vi "Data entry form.vi"(0 "Stack in":refnum<class "Stack.lvclass">, 1 "Adhesive type":string, 2 "Temperature (C)":string, 3 "Relative humidity":string, 5 "Position":dbl, 7 "Module Type":string, 9 "Module?":bool, 11 "error in (no error)":errorcluster, 12 "Operator":string, 13 "ROC version":string) -> (4 "Stack out":refnum<class "Stack.lvclass">, 8 "Cancelled?":bool, 15 "error out":errorcluster)   [LabVIEW 2021, in "Stack.lvclass"]
uses:
  Stack.lvclass
  Stack.lvclass/Stack.ctl
panel:
  in  "?":string="If blank, name automatically assigned. Check DB after submission!!!"
  in  "(optional) Module stack name (no hyphens; include 320)":string
  in  "Cancel Button":bool
  in  "Comments":string
  in  "?":string="Leave Base/Top Layer ID fields empty for dummy runs!!"
  in  "?":string="Record sensor visual inspection comments here."
  out "Sensor thickness":string
  out "BP Type":string
  out "Geometry":string
  in  "Baselayer thickness for glue dispense":dbl
  out "Resolution":string
  out "Date":string
  in  "Glue Batch":string
  in  "Component Tray ID":string
  in  "Assembly Tray ID":string
  in  "PUT ID":string
  in  "Baselayer ID":string
  in  "Toplayer ID":string
  in  "Submit":bool
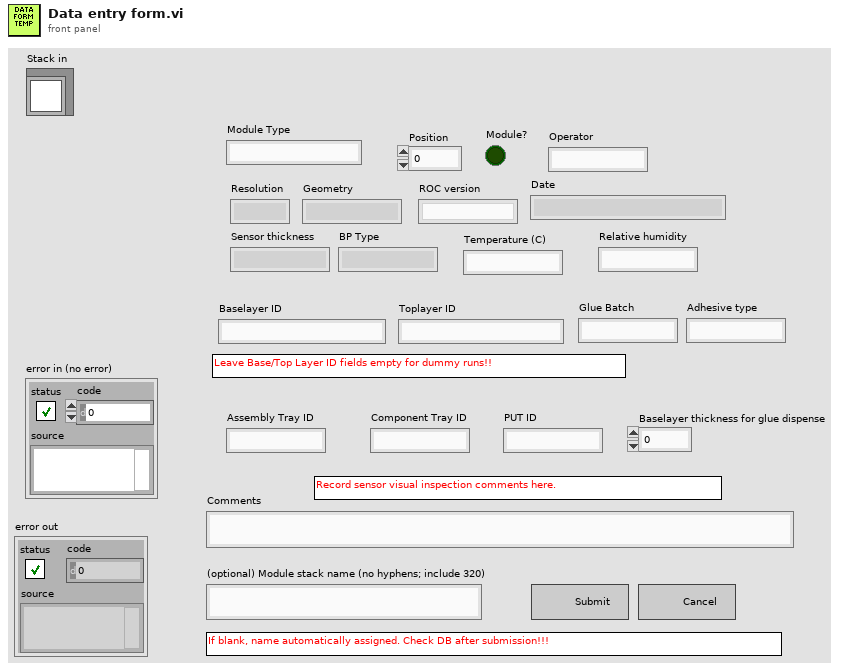
[diagram p1: front panel]
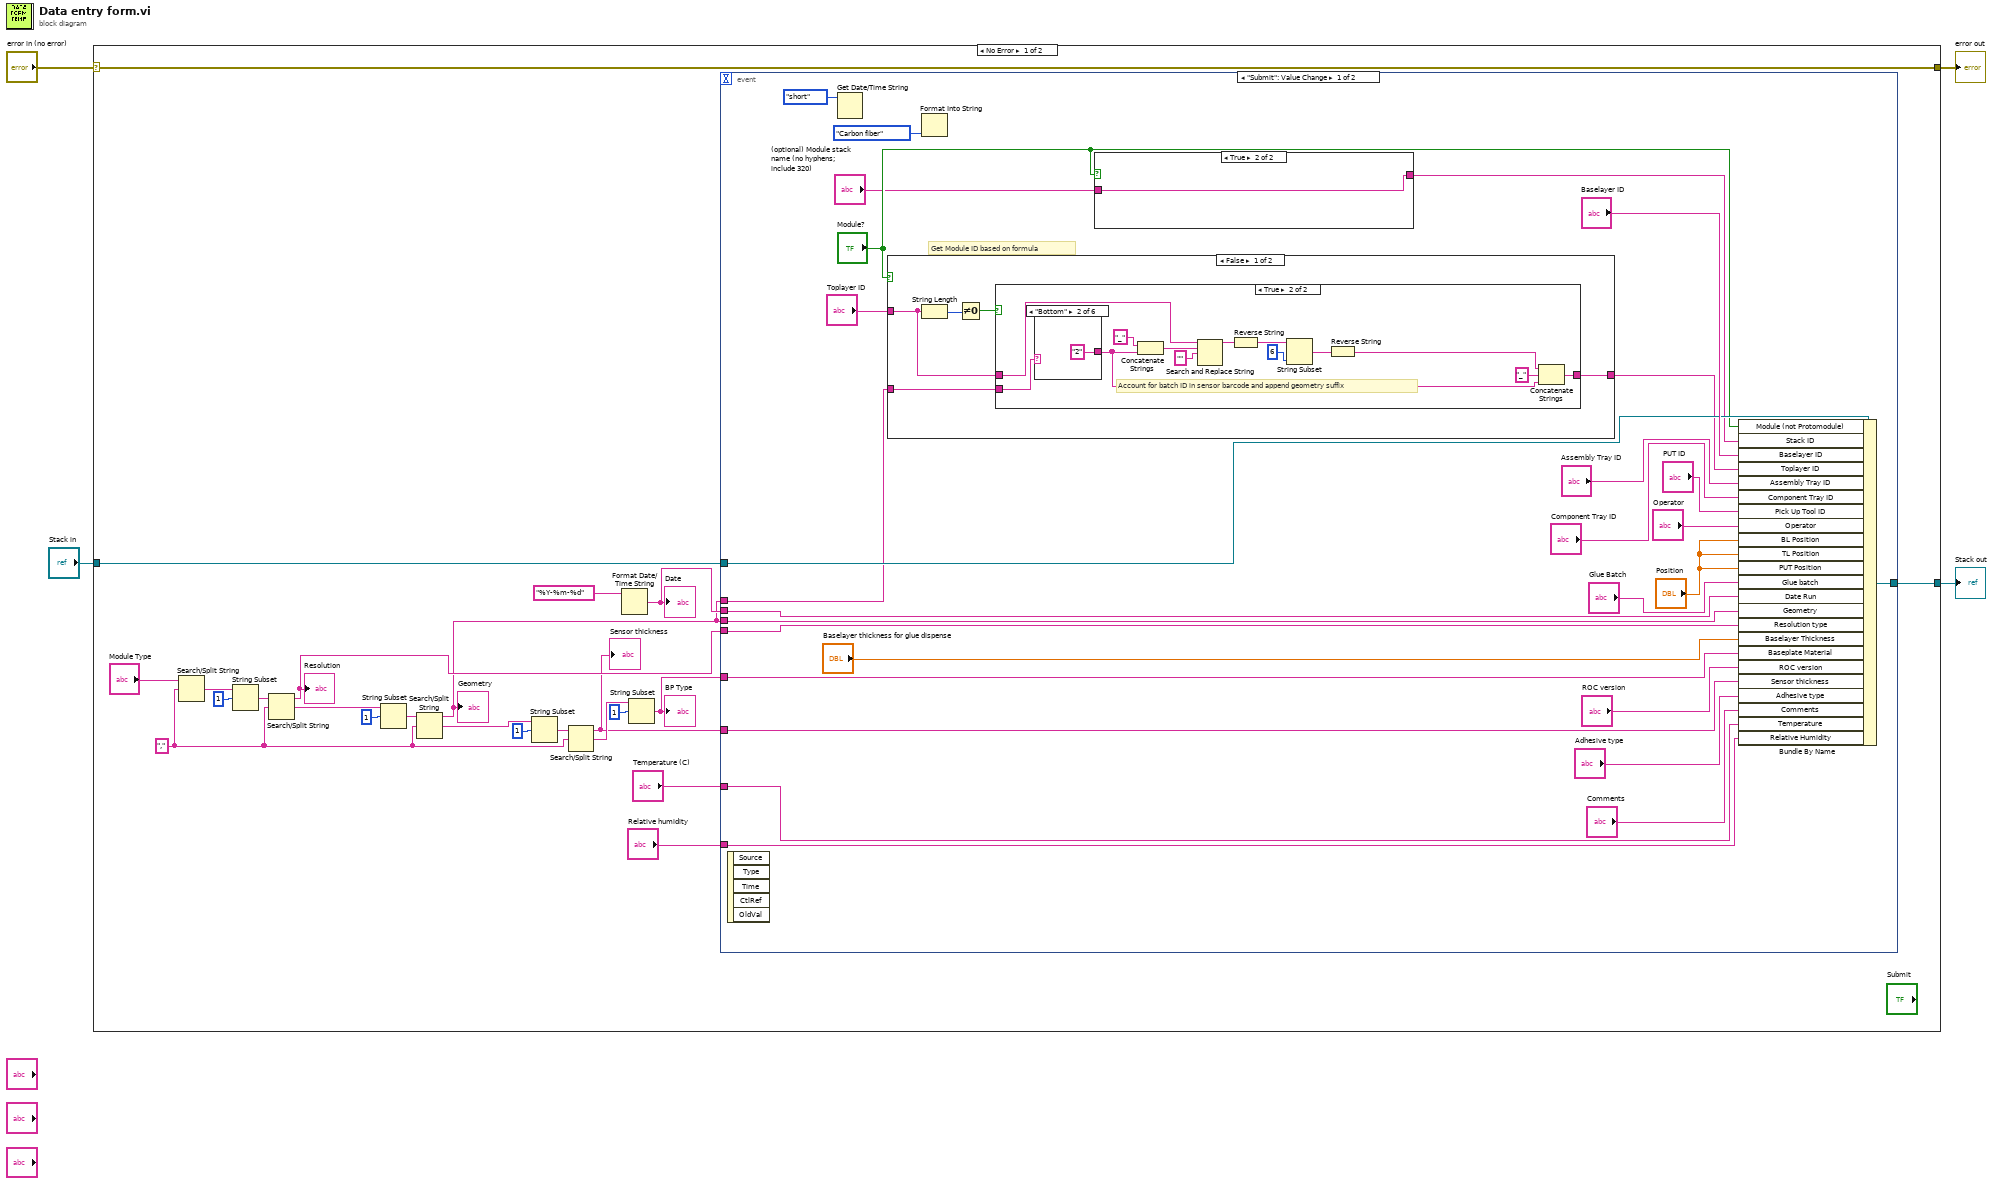
[diagram p0: block diagram]
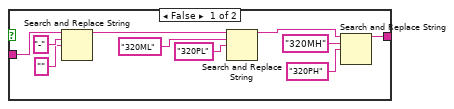
[diagram p2: hidden frame]
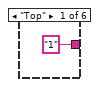
[diagram p4: hidden frame]
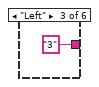
[diagram p5: hidden frame]
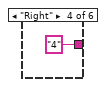
[diagram p6: hidden frame]
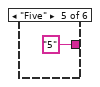
[diagram p7: hidden frame]
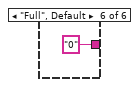
[diagram p8: hidden frame]
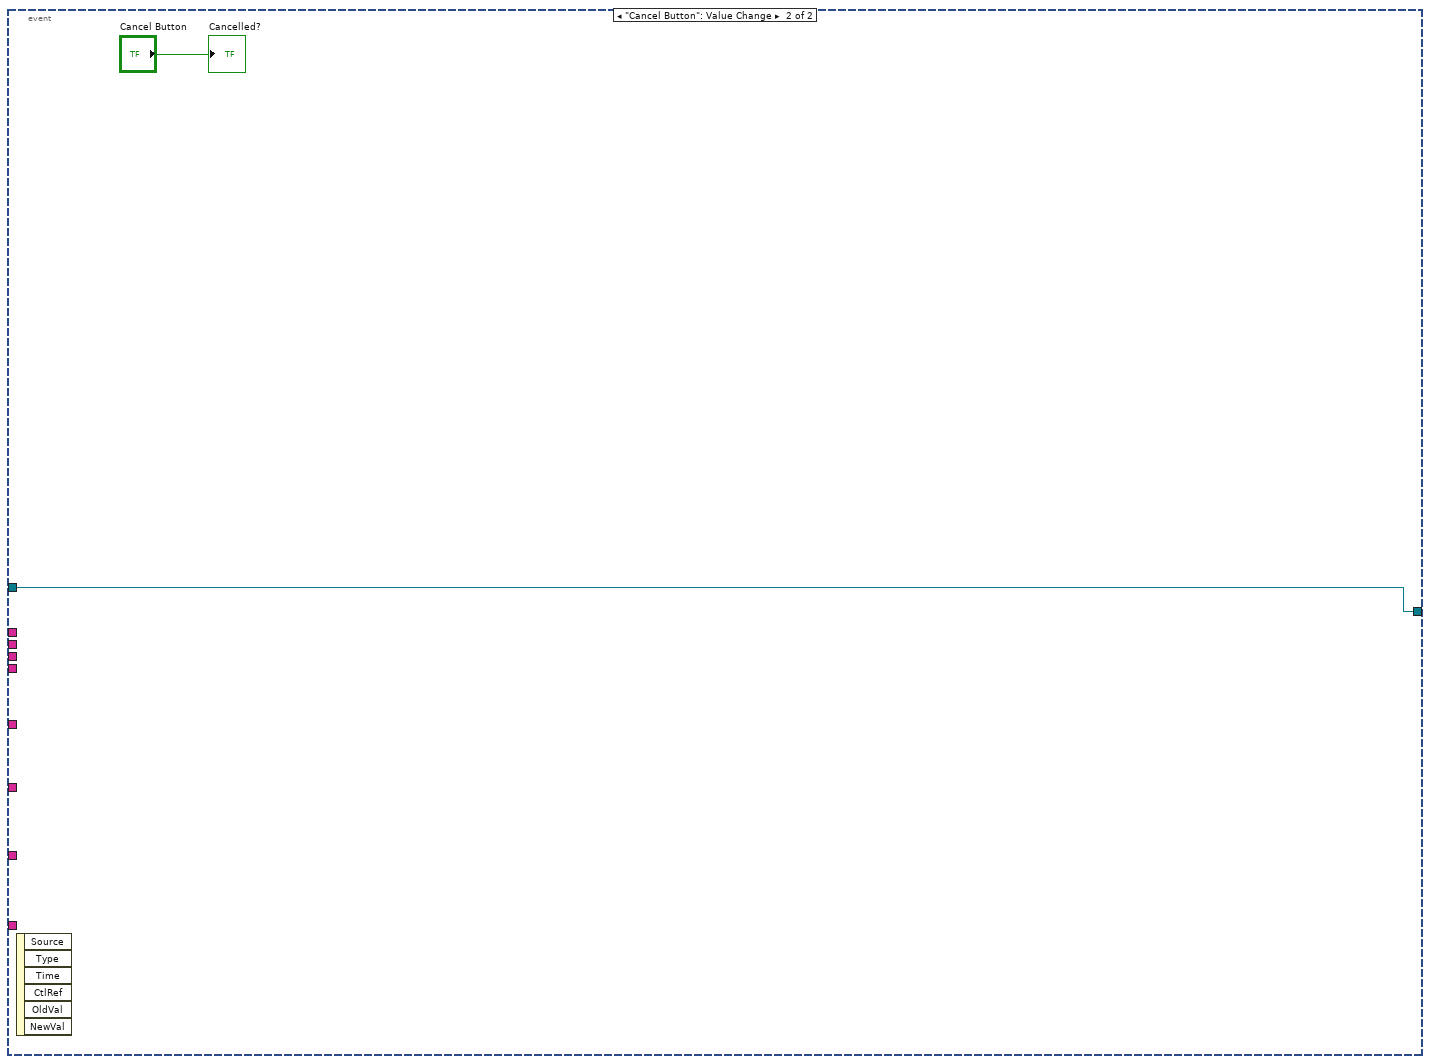
[diagram p10: hidden frame]
diagram:
  n1 = case shown="No Error" "error in (no error)" {
    selector: "error in (no error)" -> [w28 w97]
    tunnel: [w28 w97] -> w3
    tunnel: [w26 w96] -> w1
    tunnel: "Stack in" -> [w27 w96]
    frame No Error {
      w18 = "," ("search string/char (-)")
      n2 = Search/Split String(string="Module Type", search string/char (-)=w18) -> (match + rest of string=w24:string)  [unwired: 1 in, 2 out]
      n3 = String Subset(string=w24, offset (0)=1) -> (substring=w23:string)  [unwired: 1 in]
      n4 = Search/Split String(string=w23, search string/char (-)=w18) -> (substring before match=w19:string, match + rest of string=w22:string)  [unwired: 1 in, 1 out]
      "Resolution" <- w19
      n5 = String Subset(string=w22, offset (0)=1) -> (substring=w12:string)  [unwired: 1 in]
      n6 = Search/Split String(string=w12, search string/char (-)=w18) -> (substring before match=w7:string, match + rest of string=w16:string)  [unwired: 1 in, 1 out]
      "Geometry" <- w7
      n7 = String Subset(string=w16, offset (0)=1) -> (substring=w17:string)  [unwired: 1 in]
      n8 = Search/Split String(string=w17, search string/char (-)=w18) -> (substring before match=w10:string, match + rest of string=w15:string)  [unwired: 1 in, 1 out]
      "Sensor thickness" <- w10
      n9 = Format Date/Time String(time format string (%c)="%Y-%m-%d") -> (date/time string=w8:string)  [unwired: 2 in]
      "Date" <- w8
      n10 = String Subset(string=w15, offset (0)=1) -> (substring=w11:string)  [unwired: 1 in]
      "BP Type" <- w11
      n11 = event shown="[0] \"Submit\": Value Change" {
        selector: _ -> [_ _]
        dyn-events: _ -> [_ _]
        timeout: _ -> [_ _]
        tunnel: w27 -> [w54 w95]
        tunnel: [w46 w95] -> w26
        tunnel: w19 -> [w41 _]
        tunnel: w11 -> [w40 _]
        tunnel: w10 -> [w39 _]
        tunnel: w7 -> [w38 _]
        tunnel: w8 -> [w37 _]
        tunnel: w7 -> [w29 _]
        tunnel: "Temperature (C)" -> [w34 _]
        tunnel: "Relative humidity" -> [w33 _]
        event "Submit": Value Change {
          # "Get Module ID based on formula"
          n12 = event-data() -> ()  [unwired: 1 in, 5 out]
          n13 = Get Date/Time String(date format (0)=enum16{"short", "long", "abbreviated"}."short") -> ()  [unwired: 2 in, 2 out]
          n14 = case shown="False" "Module?" {
            tunnel: w29 -> [w72 _]
            tunnel: "Toplayer ID" -> [w68 w93]
            tunnel: [w71 w93] -> w35
            frame False {
              n15 = String Length(string=w68) -> (length=w70:i32)
              n16 = Not Equal To 0?(x=w70) -> (x != 0?=w69:bool)
              n17 = case shown="True" w69 {
                tunnel: w72 -> [_ w86]
                tunnel: [w73 w84] -> w71
                tunnel: w68 -> [w73 w79]
                frame False {
                }
                frame True {
                  # "Account for batch ID in sensor barcode and append geometry suffix"
                  n18 = case shown="\"Bottom\"" w86 {
                    tunnel: ["1" "2" "3" "4" "5" "0"] -> w78
                    frame "Top" {
                    }
                    frame "Bottom" {
                    }
                    frame "Left" {
                    }
                    frame "Right" {
                    }
                    frame "Five" {
                    }
                    frame "Full", Default {
                    }
                  }
                  n19 = Concatenate Strings("_" ("string"), w78) -> (w76:string)
                  n20 = Search and Replace String(input string=w79, search string=w76, replace string="" ("replace string (\"\")")) -> (result string=w74:string)  [unwired: 5 in, 3 out]
                  n21 = Reverse String(1:w74) -> (0:w83:string)
                  n22 = String Subset(string=w83, length (rest)=6 ("length (rest)")) -> (substring=w81:string)  [unwired: 1 in]
                  n23 = Reverse String(1:w81) -> (0:w80:string)
                  n24 = Concatenate Strings(w80, "_" ("string"), w78) -> (w84:string)
                }
              }
            }
            frame True {
            }
          }
          n25 = Format Into String(enum16{"CuW", "PCB", "Carbon fiber"}."Carbon fiber") -> ()  [unwired: 3 in, 2 out]
          n26 = case shown="True" "Module?" {
            tunnel: "(optional) Module stack name (no hyphens; include 320)" -> [w60 w67]
            tunnel: [w65 w67] -> w30
            frame False {
              n27 = Search and Replace String(input string=w60, search string="-", replace string="" ("replace string (\"\")")) -> (result string=w59:string)  [unwired: 5 in, 3 out]
              n28 = Search and Replace String(input string=w59, search string="320ML", replace string="320PL" ("replace string (\"\")")) -> (result string=w66:string)  [unwired: 5 in, 3 out]
              n29 = Search and Replace String(input string=w66, search string="320MH", replace string="320PH" ("replace string (\"\")")) -> (result string=w65:string)  [unwired: 5 in, 3 out]
            }
            frame True {
            }
          }
          n30 = Bundle By Name(cluster=w54, "Module (not Protomodule)"="Module?", "Stack ID"=w30, "Baselayer ID"="Baselayer ID", "Toplayer ID"=w35, "Assembly Tray ID"="Assembly Tray ID", "Component Tray ID"="Component Tray ID", "Pick Up Tool ID"="PUT ID", "Operator"="Operator", "BL Position"="Position", "TL Position"="Position", "PUT Position"="Position", "Glue batch"="Glue Batch", "Date Run"=w37, "Geometry"=w38, "Resolution type"=w41, "Baselayer Thickness"="Baselayer thickness for glue dispense", "Baseplate Material"=w40, "ROC version"="ROC version", "Sensor thickness"=w39, "Adhesive type"="Adhesive type", "Comments"="Comments", "Temperature"=w34, "Relative Humidity"=w33) -> (w46:refnum<class "Stack.lvclass">)
        }
        event "Cancel Button": Value Change {
          n31 = event-data() -> ()  [unwired: 1 in, 6 out]
          "Cancelled?" <- "Cancel Button"
        }
      }
    }
    frame Error {
    }
  }
  "error out" <- w3
  "Stack out" <- w1
